vi "Open Device.vi"(8 "error in (no error)":errorcluster, 9 "input cluster":T4={"Video Resolution"=enum."FREENECT_RESOLUTION_LOW", "Video Format"=enum."FREENECT_VIDEO_RGB", "Depth Format"=enum."FREENECT_DEPTH_11BIT", "Depth Resolution"=enum."FREENECT_RESOLUTION_LOW"}, 10 "device index":i32, 11 "Context_handle":i64) -> (0 "error out":errorcluster, 3 "handle":i64)   [LabVIEW 2015]
uses:
  Video Resolution Control.ctl
  Video Format Control.ctl
  Depth Resolution Control.ctl
  libkinect_wrapper.dll
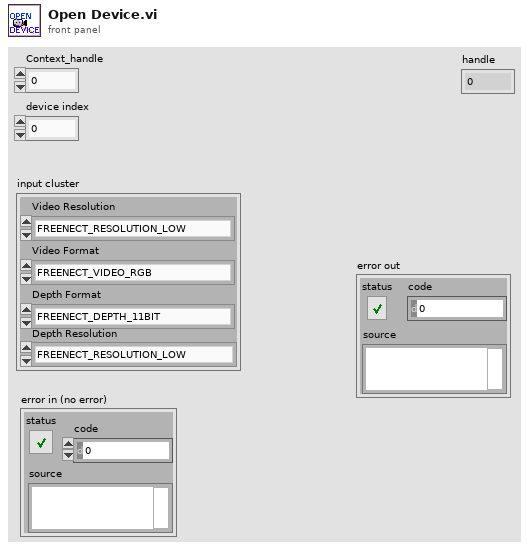
[diagram p1: front panel]
types:
  T1 = typedef "Video Resolution Control.ctl" = enum32{"FREENECT_RESOLUTION_LOW", "FREENECT_RESOLUTION_MEDIUM", "FREENECT_RESOLUTION_HIGH"}
  T2 = typedef "Video Format Control.ctl" = enum32{"FREENECT_VIDEO_RGB", "FREENECT_VIDEO_BAYER", "FREENECT_VIDEO_IR_8BIT", "FREENECT_VIDEO_IR_10BIT", "FREENECT_VIDEO_IR_10BIT_PACKED", "FREENECT_VIDEO_YUV_RGB", "FREENECT_VIDEO_YUV_RAW"}
  T3 = typedef "Depth Resolution Control.ctl" = enum16{"FREENECT_RESOLUTION_TINY", "FREENECT_RESOLUTION_LOW", "FREENECT_RESOLUTION_MEDIUM"}
  T4 = cluster{"Video Resolution":T1, "Video Format":T2, "Depth Format":enum32{"FREENECT_DEPTH_11BIT", "FREENECT_DEPTH_10BIT", "FREENECT_DEPTH_11BIT_PACKED", "FREENECT_DEPTH_10BIT_PACKED", "FREENECT_DEPTH_REGISTERED", "FREENECT_DEPTH_MM"}, "Depth Resolution":T3}
  T5 = enum32{"FREENECT_DEPTH_11BIT", "FREENECT_DEPTH_10BIT", "FREENECT_DEPTH_11BIT_PACKED", "FREENECT_DEPTH_10BIT_PACKED", "FREENECT_DEPTH_REGISTERED", "FREENECT_DEPTH_MM"}
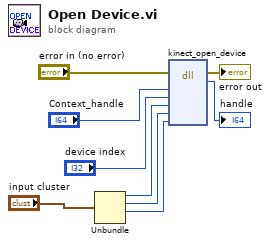
[diagram p0: block diagram]
diagram:
  n1 = Unbundle("input cluster") -> ("Video Resolution"=w3:T1, "Video Format"=w2:T2, "Depth Format"=w1:T5)  [unwired: 1 out]
  n2 = dll-call lib="libkinect_wrapper.*" fn="kinect_open_device"(error in="error in (no error)", "Context_handle"="Context_handle", "index"="device index", "video_resolution"=w3, "video_format"=w2, "depth_format"=w1) -> (error out=→"error out":errorcluster, "handle"=→"handle":i64)  [unwired: 7 in, 1 out]
